vi "Functional Imaging-Viewer events handler.vi"(8 "error in (no error)":errorcluster, 9 "NewRange":T1, 11 "Event Function":T3) -> (0 "error out":errorcluster, 3 "Event Registration Refnum":T2)   [LabVIEW 2020]
uses:
  Typedefs/Registered event names enum.ctl
  Typedefs/FuncImg-Events registration ref.ctl
  <vilib>/Utility/miscctls.llb/LVRangeTypeDef.ctl
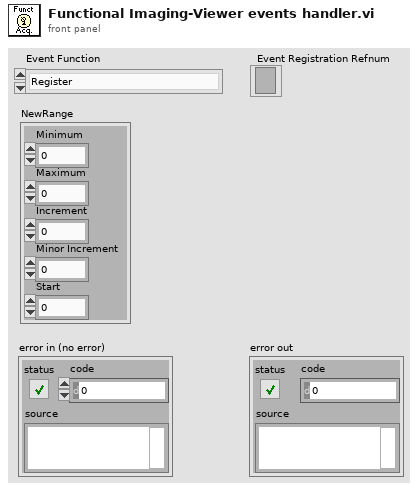
[diagram p1: front panel]
types:
  T1 = typedef "LVRangeTypeDef.ctl" = cluster{"Minimum":dbl, "Maximum":dbl, "Increment":dbl, "Minor Increment":dbl, "Start":dbl}
  T2 = typedef "FuncImg-Events registration ref.ctl" = refnum<event-registration>
  T3 = typedef "Registered event names enum.ctl" = enum16{"Register", "Load dataset in funct viewer", "Re-process data", "Export selected ROI data-full"}
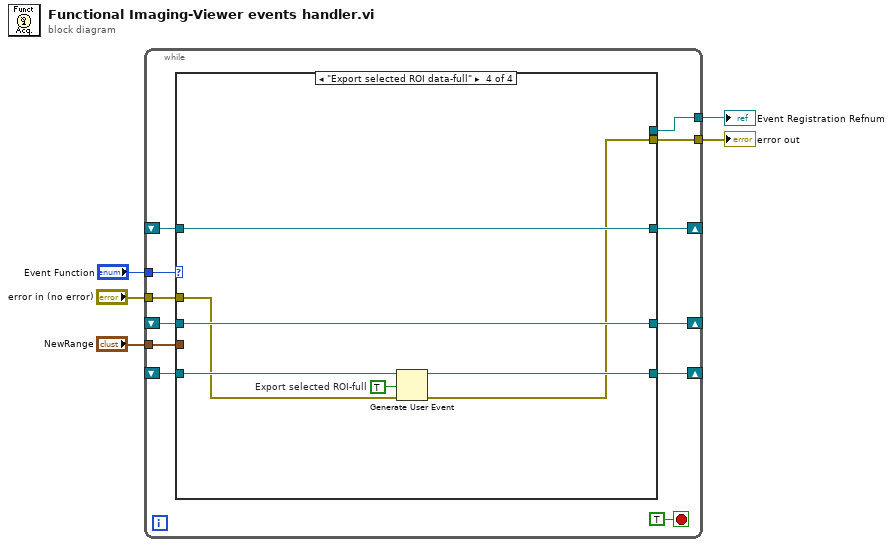
[diagram p0: block diagram]
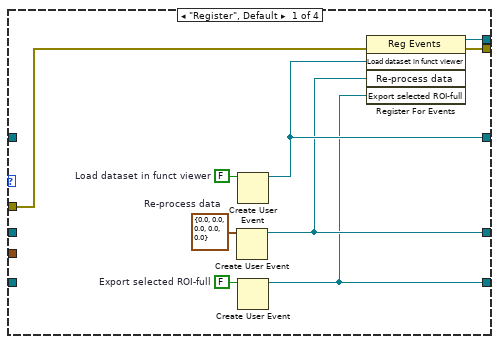
[diagram p2: hidden frame]
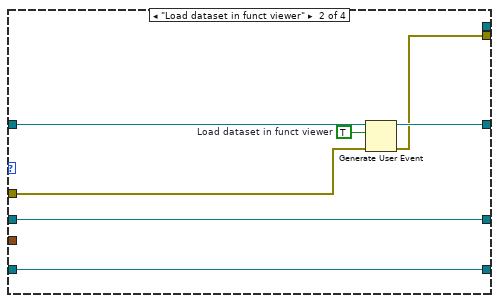
[diagram p3: hidden frame]
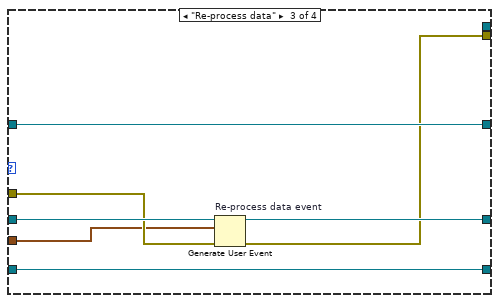
[diagram p4: hidden frame]
diagram:
  n1 = while {
    tunnel: [w8] -> w1
    tunnel: "Event Function" -> [w17]
    shift-right: [w15] -> _
    shift-left: _ -> [w14]
    shift-right: [w13] -> _
    shift-left: _ -> [w12]
    tunnel: [w11] -> w4
    tunnel: "error in (no error)" -> [w10]
    tunnel: "NewRange" -> [w9]
    shift-right: [w7] -> _
    shift-left: _ -> [w6]
    stop <- TRUE stop-if-true
    n2 = case shown="\"Export selected ROI data-full\"" w17 {
      tunnel: [w19 _ _ _] -> w8
      tunnel: [w25 w32 w40 w47] -> w15
      tunnel: w14 -> [_ w33 w40 w47]
      tunnel: [w24 w31 w38 w46] -> w13
      tunnel: w12 -> [_ w31 w39 w46]
      tunnel: [w23 w29 w36 w41] -> w11
      tunnel: w10 -> [w22 w28 w37 w42]
      tunnel: w9 -> [_ _ w35 _]
      tunnel: [w18 w27 w34 w44] -> w7
      tunnel: w6 -> [_ w27 w34 w45]
      frame "Register", Default {
        w20 = FALSE  # Export selected ROI-full
        w21 = T1 {"Minimum"=0.0, "Maximum"=0.0, "Increment"=0.0, "Minor Increment"=0.0, "Start"=0.0}  # Re-process data
        w26 = FALSE  # Load dataset in funct viewer
        n3 = Create User Event(user event datatype=w21) -> (user event=w24:refnum<user-event>)  [unwired: 1 in, 1 out]
        n4 = Create User Event(user event datatype=w26) -> (user event=w25:refnum<user-event>)  [unwired: 1 in, 1 out]
        n5 = Create User Event(user event datatype=w20) -> (user event=w18:refnum<user-event>)  [unwired: 1 in, 1 out]
        n6 = register-events(error in=w22, w25, w24, w18) -> (reference out=w19:refnum<event-registration>, error out=w23:errorcluster)  [unwired: 1 in]
      }
      frame "Load dataset in funct viewer" {
        w30 = TRUE  # Load dataset in funct viewer
        n7 = Generate User Event(user event=w33, event data cluster=w30, error in=w28) -> (user event out=w32:refnum<user-event>, error out=w29:errorcluster)  [unwired: 1 in]
      }
      frame "Re-process data" {
        n8 = Generate User Event "Re-process data event"(user event=w39, event data cluster=w35, error in=w37) -> (user event out=w38:refnum<user-event>, error out=w36:errorcluster)  [unwired: 1 in]
      }
      frame "Export selected ROI data-full" {
        w43 = TRUE  # Export selected ROI-full
        n9 = Generate User Event(user event=w45, event data cluster=w43, error in=w42) -> (user event out=w44:refnum<user-event>, error out=w41:errorcluster)  [unwired: 1 in]
      }
    }
  }
  "Event Registration Refnum" <- w1
  "error out" <- w4
